vi "PFI-28000-Utils_String Contains Any.vi"(0 "String":string, 5 "Values":string[](array[string])) -> (4 "Match":string, 6 "After Substring":string, 8 "Contains":bool)   [LabVIEW 2017, in "PFI-28000-Utils.lvlib"]
uses:
  PFI-28000-Utils.lvlib
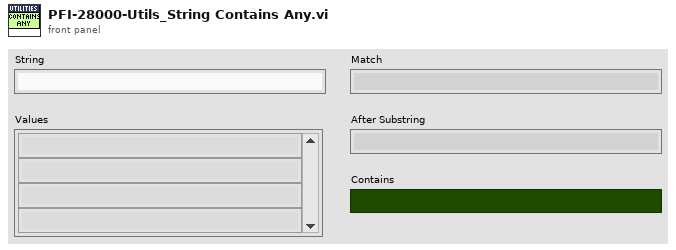
[diagram p1: front panel]
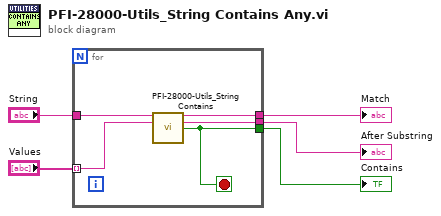
[diagram p0: block diagram]
diagram:
  n1 = for {
    tunnel: "String" -> [w10]
    tunnel: "Values" -> [w9] mode=indexing
    tunnel: [w8] -> w3
    tunnel: [w7] -> w2
    tunnel: [w6] -> w1
    stop <- w6 stop-if-true
    n2 = call "PFI-28000-Utils_String Contains.vi"("String"=w10, "Value"=w9) -> ("Match"=w8:string, "After Substring"=w7:string, "Contains"=w6:bool)  [unwired: 11 in]
  }
  "Contains" <- w1
  "After Substring" <- w2
  "Match" <- w3
